vi "Add Tab Button - Label--Const.vi"() -> (3 "Add Tab Control Label":string)   [LabVIEW 2017, in "DTacq Plot Display Library.lvlib"]
uses:
  DTacq Plot Display Library.lvlib
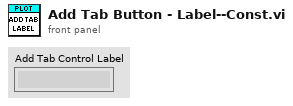
[diagram p1: front panel]
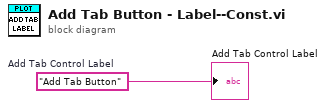
[diagram p0: block diagram]
diagram:
  w1 = "Add Tab Button"  # Add Tab Control Label
  "Add Tab Control Label" <- w1
